vi "WriteEvtConfig.vi"(8 "error in (no error)":errorcluster, 10 "Event Configuration":T1={"UTC Time 0"=timestamp(0 s since 1904-01-01), "Nominal Frequency"=60, "Reporting Rate"=60, "Fsamp"=960, "PosSeq"=FALSE} {"Reporting Rate" items=["10 FPS"=10, "12 FPS"=12, "15 FPS"=15, "20 FPS"=20, "25 FPS"=25, "30 FPS"=30, "50 FPS"=50, "60 FPS"=60]; "Nominal Frequency" items=["50 Hz"=50, "60 Hz"=60]}, 11 "RingdownPlugin in":refnum<class "RingdownPlugin.lvclass">) -> (0 "error out":errorcluster, 3 "RingdownPlugin out":refnum<class "RingdownPlugin.lvclass">)   [LabVIEW 2014, in "AppPlugins.lvlib" / "RingdownPlugin.lvclass"]
uses:
  RingdownPlugin.lvclass
  Framework/FrontPanel/TypeDefs/clEventConfig.ctl
  RingdownPlugin.lvclass/RingdownPlugin.ctl
  Accessors/Read RingdownConfig.vi
  Framework/Framework.lvlib
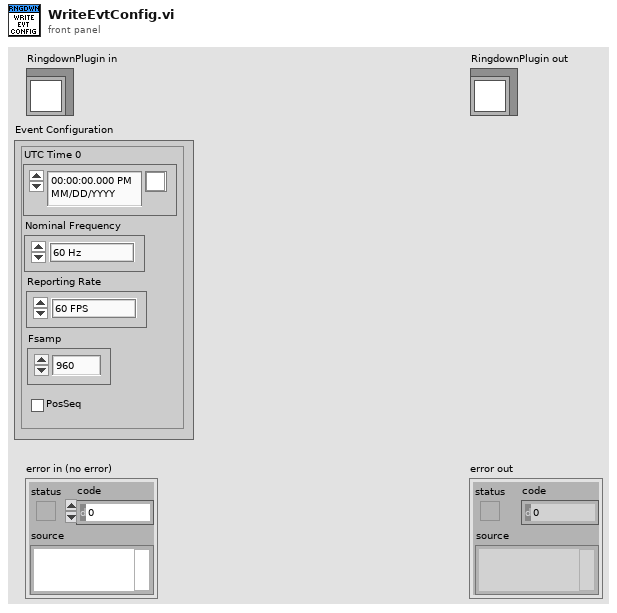
[diagram p1: front panel]
types:
  T1 = typedef "Framework.lvlib/clEventConfig.ctl" = cluster{"UTC Time 0":timestamp, "Nominal Frequency":u16, "Reporting Rate":u16, "Fsamp":u32, "PosSeq":bool}
  T2 = typedef "AppPlugins.lvlib/RingdownPlugin.lvclass/RingdownConfig.ctl" = cluster{"Config":cluster{"Addmod":i32, "Scalmod":i32, "Lpocon":i32, "Pircon":i32, "Dmodes":i32, "Lpmcon":u16, "Lpacon":u16, "Fbcon":u16, "Ordcon":i32, "Trimre":dbl, "Ftrimh":dbl, "Ftriml":dbl}, "Window":cluster{"StOffset":i32, "EndOffset":i32, "Length":i32}, "V index":i32, "I index":i32, "PosSeq":bool}
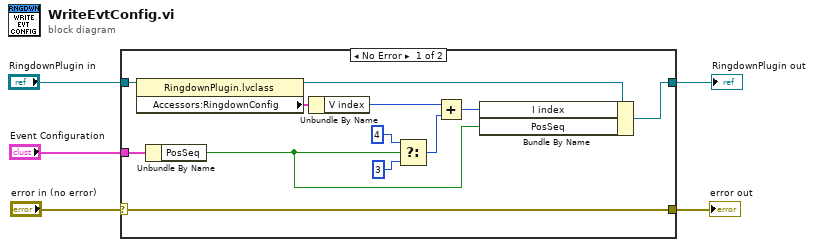
[diagram p0: block diagram]
diagram:
  n1 = case shown="No Error" "error in (no error)" {
    selector: "error in (no error)" -> [w7 w18]
    tunnel: "RingdownPlugin in" -> [w16 w19]
    tunnel: [w8 w19] -> w3
    tunnel: [w7 w18] -> w2
    tunnel: "Event Configuration" -> [w17 _]
    frame No Error {
      n2 = property class="RingdownPlugin.lvclass"(reference=w16) -> (reference out=w10:refnum<class "RingdownPlugin.lvclass">, "Accessors:RingdownConfig"=w15:T2)  [unwired: 1 in, 1 out]
      n3 = Unbundle By Name(w17) -> ("PosSeq"=w6:bool)
      n4 = Unbundle By Name(w15) -> ("V index"=w11:i32)
      n5 = Select(t=4, s=w6, f=3) -> (s? t:f=w12:i32)
      n6 = Add(x=w11, y=w12) -> (x+y=w9:i32)
      n7 = Bundle By Name(cluster=w10, "I index"=w9, "PosSeq"=w6) -> (w8:refnum<class "RingdownPlugin.lvclass">)
    }
    frame Error {
    }
  }
  "error out" <- w2
  "RingdownPlugin out" <- w3
